vi "TC_GetFromRefArray.vi"(5 "arrayIn":T1, 11 "NameToFind":string) -> (0 "arrayOut":T1, 3 "refArray":refnum<vi>[](array[refnum]))   [LabVIEW 2017]
uses:
  RefArray.ctl
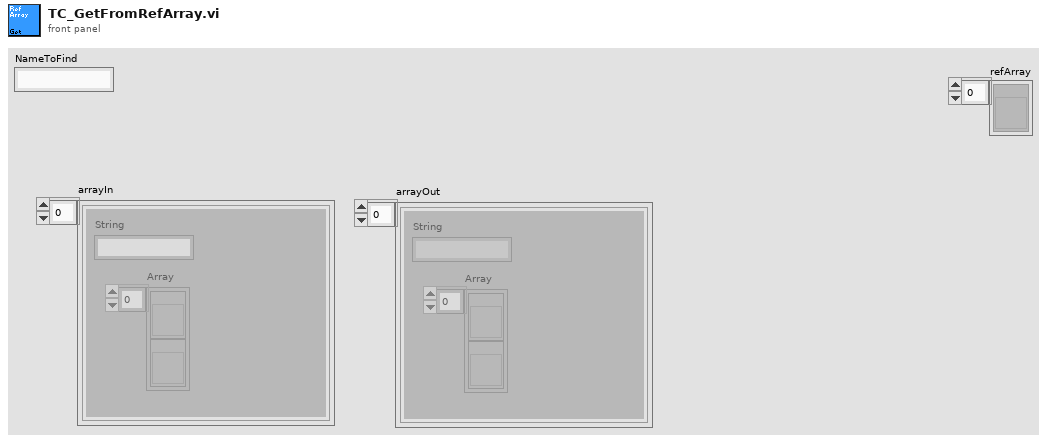
[diagram p1: front panel]
types:
  T1 = typedef "RefArray.ctl" = cluster{"String":string, "Array":refnum<vi>[]}[]
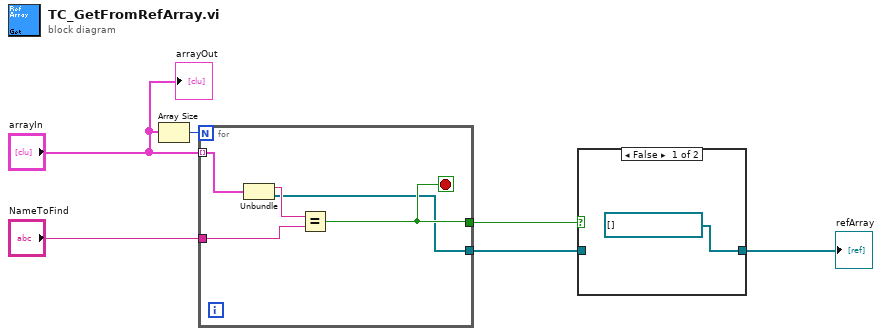
[diagram p0: block diagram]
diagram:
  n1 = Array Size(array="arrayIn") -> (size(s)=w5:i32)
  n2 = for {
    N: w5 -> [_]
    tunnel: "NameToFind" -> [w9]
    tunnel: "arrayIn" -> [w11] mode=indexing
    tunnel: [w8] -> w2
    tunnel: [w7] -> w1
    stop <- w8 stop-if-true
    n3 = Unbundle(w11) -> ("String"=w10:string, "Array"=w7:refnum<vi>[])
    n4 = Equal?(x=w10, y=w9) -> (x = y?=w8:bool)
  }
  n5 = case shown="False" w2 {
    tunnel: w1 -> [_ w13]
    tunnel: [refnum<vi>[] [] ("refArray") w13] -> w3
    frame False {
    }
    frame True {
    }
  }
  "refArray" <- w3
  "arrayOut" <- "arrayIn"
